vi "DePew_3rd_excersize1_11-29-16.vi"   [LabVIEW 2014, in "Exersize 1.lvrbt"]
uses:
  Exersize 1.lvrbt
  <vilib>/NXT/Dual Mode Library/Display/drawText.vi
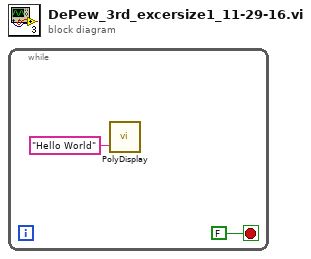
[diagram p0: block diagram]
diagram:
  n1 = while {
    stop <- FALSE stop-if-true
    n2 = call-poly <vilib>:"PolyDisplay.vi"("Text"="Hello World") -> ()  [unwired: 3 in, 1 out]
  }
